vi "Shutdown.vi"(8 "error in (no error)":errorcluster, 11 "Framework in":refnum<class "Framework.lvclass">) -> (0 "error out":errorcluster, 3 "Framework out":refnum<class "Framework.lvclass">)   [LabVIEW 2017, in "Data Sharing Framework Core.lvlib" / "Data Sharing Framework Engine.lvlib" / "Framework.lvclass"]
uses:
  Framework.lvclass
  Framework.lvclass/Framework.ctl
  Internal/Transceiver/Transceiver/Transceiver.lvclass
  Plugin/Plugin.lvclass
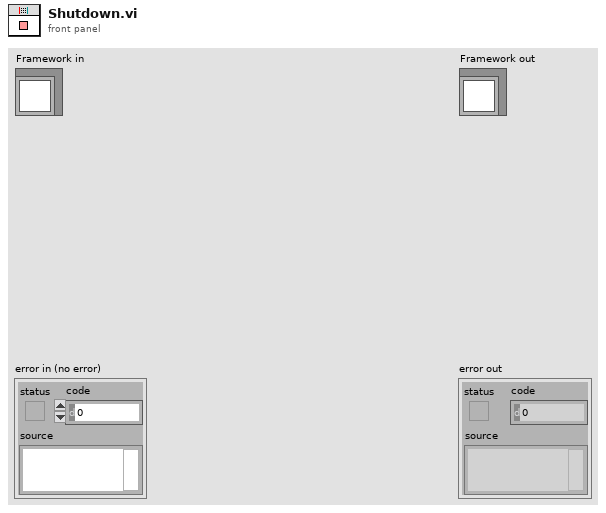
[diagram p1: front panel]
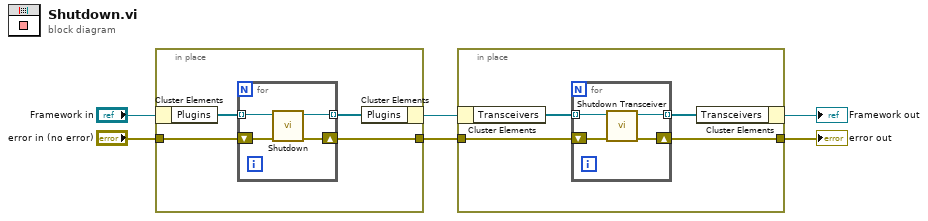
[diagram p0: block diagram]
diagram:
  n1 = in-place {
    in-place-border: "error in (no error)" -> [w10]
    in-place-border: [w9] -> w4
    n2 = in-place-cluster #1("Framework in") -> ("Plugins"=w8:refnum<class "Plugin.lvclass">[])
    n3 = for {
      tunnel: w8 -> [w11] mode=indexing
      tunnel: [w12] -> w7 mode=indexing
      shift-right: [w13] -> w9
      shift-left: w10 -> [w14]
      n4 = call "Shutdown.vi"("error in (no error)"=w14, "Plugin in"=w11) -> ("error out"=w13:errorcluster, "Plugin out"=w12:refnum<class "Plugin.lvclass">)  [unwired: 8 in]
    }
    n5 = in-place-cluster #1("Plugins"=w7) -> (w3:refnum<class "Framework.lvclass">)
  }
  n6 = in-place {
    in-place-border: w4 -> [w18]
    in-place-border: [w17] -> w2
    n7 = in-place-cluster #2(w3) -> ("Transceivers"=w16:refnum<class "Transceiver.lvclass">[])
    n8 = for {
      tunnel: w16 -> [w22] mode=indexing
      shift-right: [w20] -> w17
      shift-left: w18 -> [w21]
      tunnel: [w19] -> w15 mode=indexing
      n9 = call-dynamic "Shutdown Transceiver.vi"("error in (no error)"=w21, "Transceiver in"=w22) -> ("error out"=w20:errorcluster, "Transceiver out"=w19:refnum<class "Transceiver.lvclass">)  [unwired: 8 in]
    }
    n10 = in-place-cluster #2("Transceivers"=w15) -> (→"Framework out":refnum<class "Framework.lvclass">)
  }
  "error out" <- w2
